vi "error handler.vi"(4 "status array":bool[](array[boolean]), 5 "status":T1, 6 "poll response":i16, 7 "GPIB in":string="18") -> (0 "error occurred":bool, 1 "error list":T2(ring), 3 "GPIB out":string="18")   [LabVIEW 2015]
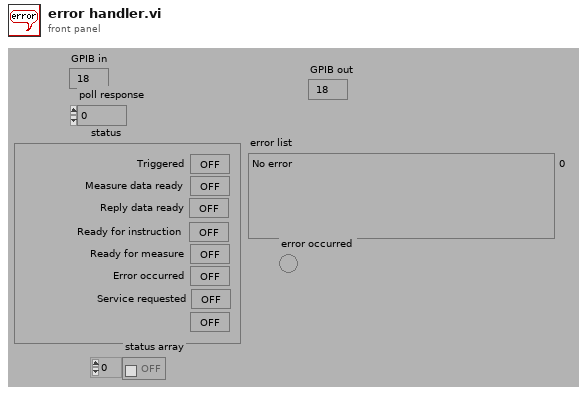
[diagram p1: front panel]
types:
  T1 = cluster{"Triggered":bool, "Measure data ready":bool, "Reply data ready":bool, "Ready for instruction":bool, "Ready for measure":bool, "Error occurred":bool, "Service requested":bool, "Power on (no instructions sent yet)":bool}
  T2 = enum16{"No error", "HP 8452A Error 1 CPU This error indicates that the instrument has experienced an intermittent CPU error.", "HP 8452A Error 2 ROM This error indicates that the instrument has experienced an intermittent ROM error.", "HP 8452A Error 3 RAM This error indicates that the instrument has experienced an intermittent RAM error.", "HP 8452A Error 4 Multiplier This error indicates that the instrument has experienced an intermittent hardware multiplier error.", "HP 8452A Error 5 Communication  This error indicates that the instrument has experienced an intermittent communication board error.", "HP 8452A Error 6 Microcontroller  This error indicates that the instrument has experienced an intermittent 8051 microcontroller error.", "HP 8452A Error 7 Interrupt This error indicates that the instrument has experienced an intermittent nonrecoverable interrupt error.", "HP 8452A Error 8 Cover Off  This error is not relevant for option #003.  This error indicates that the instrument has discovered that its cover has been removed. As a result, the instrument has turned off its deuterium lamp as a safety precaution. Before ", "HP 8452A Error 9 ADC This error indicates that the instrument has discovered that its analog to digital converter is in error.", "HP 8452A Error 10 Lamp This error indicates that the instrument has discovered that the deuterium lamp has failed to light. This could be due to an old or broken lamp.", "HP 8452A Error 11 No Light This error indicates that the instrument has been unable to detect enough light on its detector diodes to render accurate readings. Possible causes include: the light path being blocked, the shutter being stuck closed, or a filt", "HP 8452A Error 12 Leaky Diodes This error indicates that the instrument has detected one or more leaky diodes in its diode array.", "HP 8452A Error 13 No Gain This error indicates that the instrument has experienced incorrect gain amplifier response.", "HP 8452A Error 14 Diode Saturation  This error indicates that the instrument has experienced gain amplifier saturation even at the lowest gain setting on one or more diodes. This implies that too much light is being received by the diode array.", "HP 8452A Error 15 Not Enough Light  This error indicates that one or more diodes does not have enough dark current intensity. This is most often caused by an obstruction in the light path such as a filter.  It can also be caused by residual sample left in", "HP 8452A Error 15 unknown  (you should never see this error code!)", "HP 8452A Error 17 Interrupts This error indicates that the instrument has experienced a CPU interrupt that it did not expect.", "HP 8452A Error 18 Measurement  This error indicates that the instrument is generating measurement data faster than the controller is accepting. Generally this results from the measurement repeat cycle being to short and therefore occurs during repeated ti", "HP 8452A Error 19 Instruction This error indicates that the instrument was unable to recognize the most recent instruction sent to it.", "HP 8452A Error 20 Parameter This error indicates that the instrument has detected an error in the parameter list that accompanied the most recent instruction.", "HP 8452A Error 21 Range This error indicates that the instrument has detected an error in the value of a parameter that accompanied the most recent instruction.", "HP 8452A Error 22 Output Full This error indicates that the instrument has received a second instruction that generates information (reply or measurement data) before the previous information has been read.", "HP 8452A Error 23 Runtime  This error indicates that the instrument has detected a run time error such as the request for a measurement without first taking a reference measurement.", "HP 8452A Error 24 Instr Rejected  This error indicates that the instrument has determined that the most recent instruction is not acceptable given its current state.", "HP 8452A Error 25 Shutter Time This error indicates that the instrument has determined that there is not enough time to perform shutter processing with the current measurement parameters.", "HP 8452A Error 26 Transport Interface  This error indicates that the instrument has received an instruction that was to perform some type of Multicell Transport operation but that the transport accessory interface is not installed.", "HP 8452A Error 27 Transport Cable  This error indicates that HP 8452A has received an instruction that was to perform some type of Multicell Transport operation but that the transport cable is no longer installed.", "HP 8452A Error 28 Transport Movement  This error indicates that HP 8452A has received an instruction that was to perform some type of Multicell Transport operation but that the transport processor took too long to complete the operation and therefore time", "HP 8452A Error 28 unknown  (you should never see this error code!)", "HP 8452A Error 30 Command This error indicates that HP 8452A has detected a firmware or some other part of the processor board is not working.", "HP 8452A Error 31 Input Output  This error indicates that HP 8452A has detected an input or output error probably in the processor firmware or hardware."}
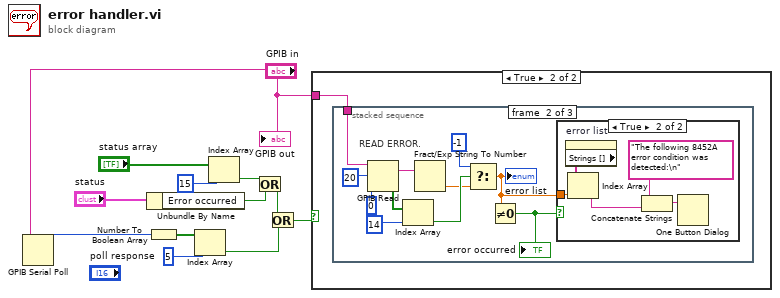
[diagram p0: block diagram]
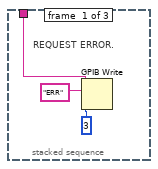
[diagram p3: hidden frame]
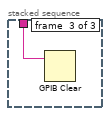
[diagram p5: hidden frame]
diagram:
  n1 = GPIB Serial Poll(0:"GPIB in") -> (2:w1:i16)  [unwired: 1 in, 2 out]
  n2 = Unbundle By Name("status") -> ("Error occurred"=w7:bool)
  n3 = Number To Boolean Array(number=w1) -> (Boolean array=w9:bool[])
  n4 = Index Array(array=w9, index=5) -> (element=w6:bool)
  n5 = Index Array(array="status array", index=15) -> (element=w8:bool)
  n6 = Or(x=w8, y=w7) -> (x .or. y?=w5:bool)
  n7 = Or(x=w5, y=w6) -> (x .or. y?=w4:bool)
  n8 = case shown="True" w4 {
    tunnel: "GPIB in" -> [_ w13]
    frame False {
    }
    frame True {
      n9 = stacked-sequence {
        tunnel: w13 -> [w14 w19 w33]
        frame #0 {
          # "REQUEST ERROR."
          n10 = GPIB Write(0:w14, 1:"ERR", 2:3) -> ()  [unwired: 2 in, 2 out]
        }
        frame #1 {
          # "READ ERROR."
          n11 = GPIB Read(0:w19, 1:20, 2:0) -> (5:w22:string, 6:w23:bool[])  [unwired: 2 in, 1 out]
          n12 = Index Array(array=w23, index=14) -> (element=w26:bool)
          n13 = Fract/Exp String To Number(string=w22) -> (number=w25:dbl)  [unwired: 3 in, 1 out]
          n14 = Select(t=-1, s=w26, f=w25) -> (s? t:f=w18:dbl)
          "error list" <- w18
          n15 = Not Equal To 0?(x=w18) -> (x != 0?=w17:bool)
          "error occurred" <- w17
          n16 = case shown="True" w17 {
            tunnel: w18 -> [_ w28]
            frame False {
            }
            frame True {
              n17 = property on="error list" class="Enum (strict)"() -> ("Strings []"=w29:string[])  [unwired: 2 in, 2 out]
              n18 = Index Array(array=w29, index=w28) -> (element=w30:string)
              n19 = Concatenate Strings("The following 8452A error condition was detected:\n", w30) -> (w32:string)
              n20 = One Button Dialog(message=w32) -> ()  [unwired: 1 in, 1 out]
            }
          }
        }
        frame #2 {
          n21 = GPIB Clear(3:w33) -> ()  [unwired: 1 in, 2 out]
        }
      }
    }
  }
  "GPIB out" <- "GPIB in"
